vi "Drive Direction.vi"(6 "Wheel DevRef":T1={"DeviceStatus"={"status"=FALSE, "code"=0, "source"=""}, "Type"=enum."PWM", "PWM"={"PWM Channel"=enum."Invalid", "DeadBand"={"Name"="", "maxPositivePwm"=0, "minPositivePwm"=0, "centerPwm"=0, "maxNegativePwm"=0, "minNegativePwm"=0, "angularRange"=0}}, "CAN"={"Device Number"=0, "SetOutput VI Ref"=variant(refnum<vi> refnum), "GetOutput VI Ref"=variant(refnum<vi> refnum), "Enable VI Ref"=variant(refnum<vi> refnum), "Disable VI Ref"=variant(refnum<vi> refnum), "Data"=variant}, "Invert"=FALSE}, 7 "Swerve DevRef":T1={"DeviceStatus"={"status"=FALSE, "code"=0, "source"=""}, "Type"=enum."PWM", "PWM"={"PWM Channel"=enum."PWM 1", "DeadBand"={"Name"="", "maxPositivePwm"=0, "minPositivePwm"=0, "centerPwm"=0, "maxNegativePwm"=0, "minNegativePwm"=0, "angularRange"=0}}, "CAN"={"Device Number"=0, "SetOutput VI Ref"=variant(enum8{"Percent VBus", "Current", "Speed", "Position", "Voltage"} enum."Percent VBus"), "GetOutput VI Ref"=variant(refnum<k1> refnum), "Enable VI Ref"=variant(dbl 12.0), "Disable VI Ref"=variant(enum8{"Percent VBus", "Speed", "Position", "Slave", "Unchanged / Invalid", "Voltage Compensation", "Current", "Motion Profile"} enum."Percent VBus"), "Data"=variant}, "Invert"=FALSE}, 8 "error in":errorcluster, 9 "Wheel Power":dbl format="%#_13g", 10 "Desired direction (radians)":dbl=6.283185307179586 format="%#_13g") -> (0 "error out":errorcluster, 1 "Setpoint":dbl, 2 "Wheel Speed":dbl, 3 "Swerve Speed":dbl, 4 "Reverse?":bool)   [LabVIEW 2016]
uses:
  <vilib>/Rock Robotics/WPI/MotorControl/WPI_MotorControlDeviceRef.ctl
  <vilib>/Rock Robotics/WPI/MotorControl/WPI_MotorControlType.ctl
  <vilib>/Rock Robotics/SystemInterfaces/DIO/FPGA_DIOPWMChannel.ctl
  <vilib>/Rock Robotics/WPI/PWM/WPI_PWMDeadband.ctl
  Main/Robot Global Data.vi
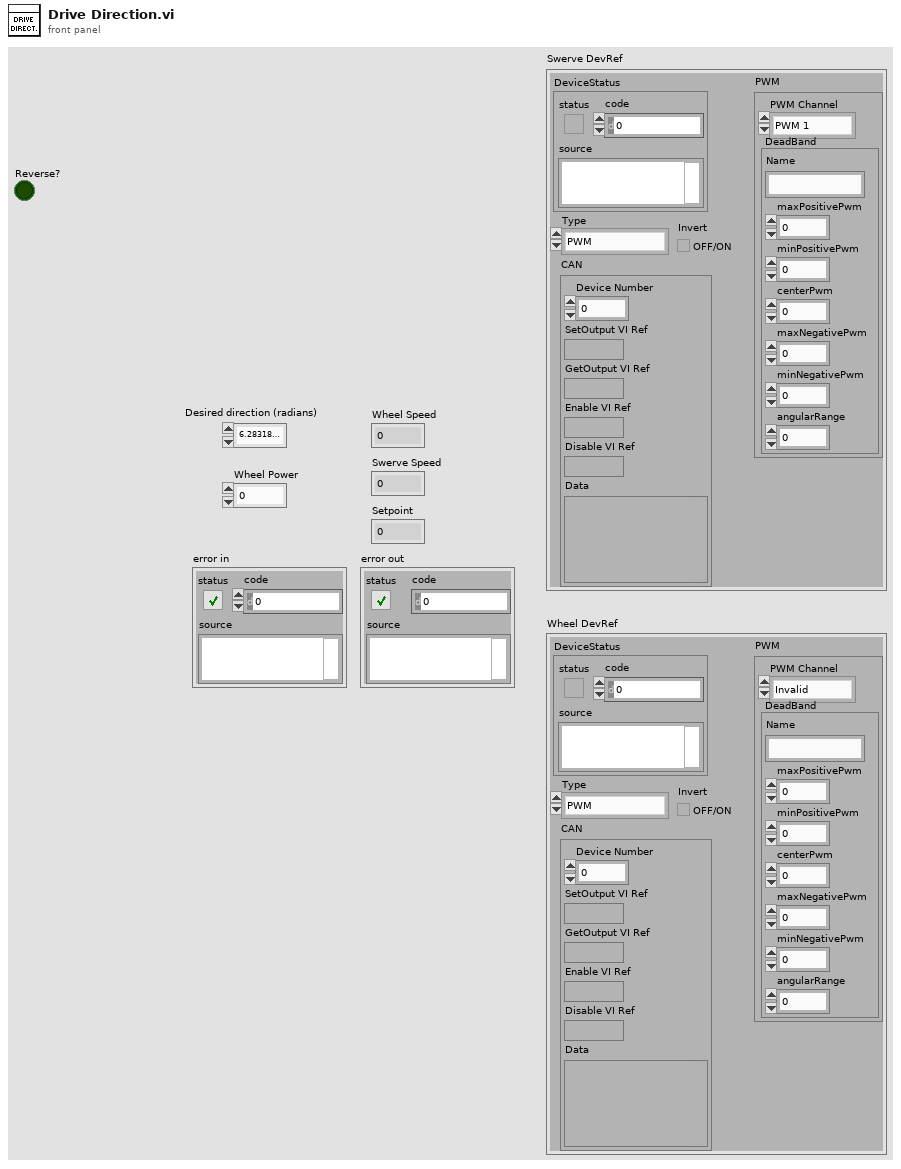
[diagram p1: front panel]
types:
  T1 = typedef "WPI_MotorControlDeviceRef.ctl" = cluster{"DeviceStatus":errorcluster, "Type":T2, "PWM":cluster{"PWM Channel":T3, "DeadBand":T4}, "CAN":cluster{"Device Number":u8, "SetOutput VI Ref":variant, "GetOutput VI Ref":variant, "Enable VI Ref":variant, "Disable VI Ref":variant, "Data":variant}, "Invert":bool}
  T2 = typedef "WPI_MotorControlType.ctl" = enum16{"PWM", "CAN"}
  T3 = typedef "FPGA_DIOPWMChannel.ctl" = enum8{"PWM 0", "PWM 1", "PWM 2", "PWM 3", "PWM 4", "PWM 5", "PWM 6", "PWM 7", "PWM 8", "PWM 9", "PWM MXP 0", "PWM MXP 1", "PWM MXP 2", "PWM MXP 3", "PWM MXP 4", "PWM MXP 5", "PWM MXP 6", "PWM MXP 7", "PWM MXP 8", "PWM MXP 9", "Invalid"}
  T4 = typedef "WPI_PWMDeadband.ctl" = cluster{"Name":string, "maxPositivePwm":i32, "minPositivePwm":i32, "centerPwm":i32, "maxNegativePwm":i32, "minNegativePwm":i32, "angularRange":u16}
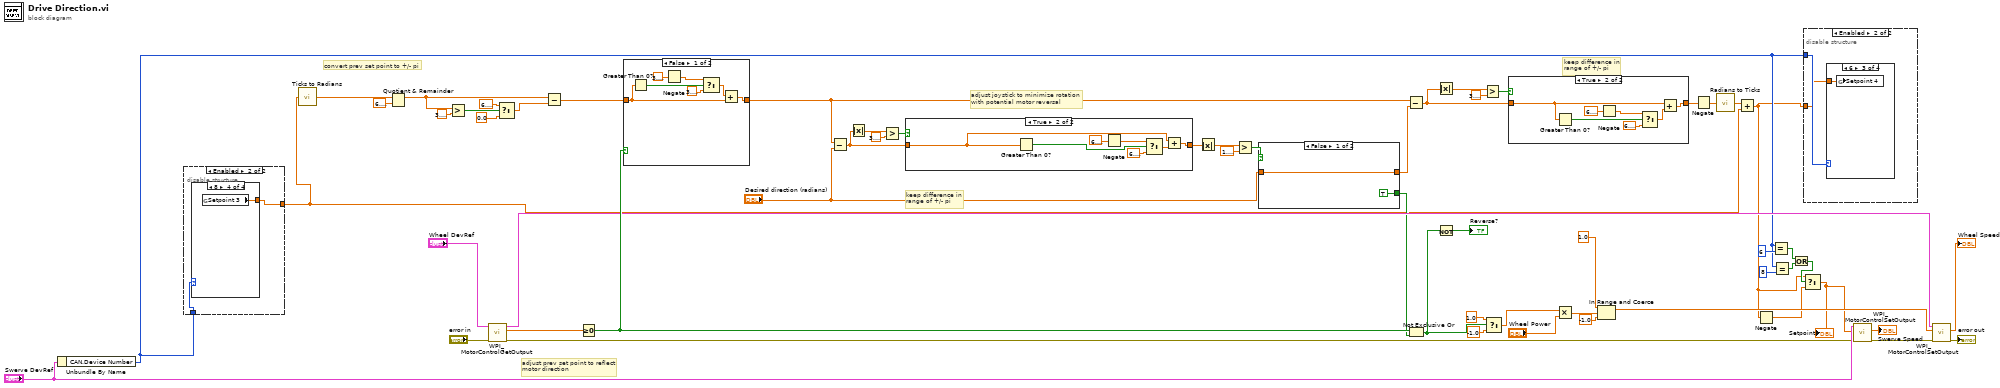
[diagram p0: block diagram]
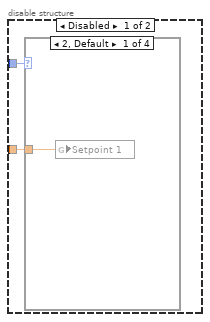
[diagram p2: hidden frame]
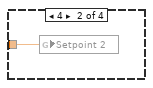
[diagram p3: hidden frame]
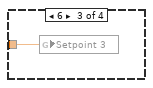
[diagram p4: hidden frame]
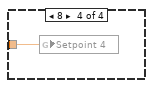
[diagram p5: hidden frame]
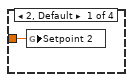
[diagram p6: hidden frame]
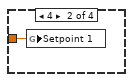
[diagram p7: hidden frame]
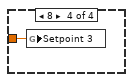
[diagram p8: hidden frame]
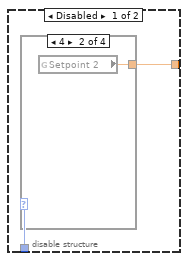
[diagram p9: hidden frame]
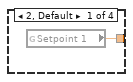
[diagram p10: hidden frame]
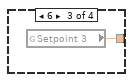
[diagram p11: hidden frame]
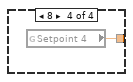
[diagram p12: hidden frame]
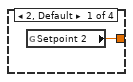
[diagram p13: hidden frame]
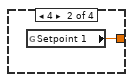
[diagram p14: hidden frame]
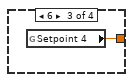
[diagram p15: hidden frame]
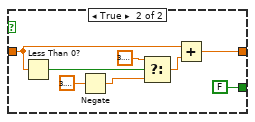
[diagram p17: hidden frame]
diagram:
  # "keep difference in\nrange of +/- pi"
  # "adjust joystick to minimize rotation\nwith potential motor reversal"
  # "keep difference in\nrange of +/- pi"
  # "adjust prev set point to reflect\nmotor direction"
  # "convert prev set point to +/- pi"
  n1 = Unbundle By Name("Swerve DevRef") -> ("CAN.Device Number"=w2:u8)
  n2 = disable-structure shown="Enabled" {
    disable-tunnel: w2 -> [w61 w67]
    disable-tunnel: [w60 w66] -> w22
    frame Disabled {
      n3 = case shown="4" w61 {
        tunnel: [w62 w63 w64 w65] -> w60
        frame 2, Default {
          n4 = global read "Robot Global Data.vi" "Setpoint 1"() -> (w62:dbl)
        }
        frame 4 {
          n5 = global read "Robot Global Data.vi" "Setpoint 2"() -> (w63:dbl)
        }
        frame 6 {
          n6 = global read "Robot Global Data.vi" "Setpoint 3"() -> (w64:dbl)
        }
        frame 8 {
          n7 = global read "Robot Global Data.vi" "Setpoint 4"() -> (w65:dbl)
        }
      }
    }
    frame Enabled {
      n8 = case shown="8" w67 {
        tunnel: [w68 w69 w70 w71] -> w66
        frame 2, Default {
          n9 = global read "Robot Global Data.vi" "Setpoint 2"() -> (w68:dbl)
        }
        frame 4 {
          n10 = global read "Robot Global Data.vi" "Setpoint 1"() -> (w69:dbl)
        }
        frame 6 {
          n11 = global read "Robot Global Data.vi" "Setpoint 4"() -> (w70:dbl)
        }
        frame 8 {
          n12 = global read "Robot Global Data.vi" "Setpoint 3"() -> (w71:dbl)
        }
      }
    }
  }
  n13 = call "Ticks to Radians.vi"("Ticks"=w22) -> ("Radians"=w47:dbl)
  n14 = Quotient & Remainder(x=w47, y=6.283185307179586) -> (x-y*floor(x/y)=w53:dbl)  [unwired: 1 out]
  n15 = Greater?(x=w53, y=3.141592653589793) -> (0:w57:bool)
  n16 = call <vilib>:"WPI_MotorControlGetOutput.vi"("error in"="error in", "MotorControlDevRef"="Wheel DevRef") -> ("error out"=w20:errorcluster, "Output"=w41:dbl, "MotorControlDevRef"=w40:T1)  [unwired: 7 in]
  n17 = Select(t=6.283185307179586, s=w57, f=0.0) -> (s? t:f=w54:dbl)
  n18 = Subtract(x=w53, y=w54) -> (x-y=w49:dbl)
  n19 = Greater Or Equal To 0?(x=w41) -> (x >= 0?=w48:bool)
  n20 = case shown="False" w48 {
    tunnel: w49 -> [w73 w79]
    tunnel: [w72 w79] -> w35
    frame False {
      n21 = Greater Than 0?(x=w73) -> (x > 0?=w78:bool)
      n22 = Negate(x=3.141592653589793) -> (-x=w77:dbl)
      n23 = Select(t=w77, s=w78, f=3.141592653589793) -> (s? t:f=w74:dbl)
      n24 = Add(x=w74, y=w73) -> (x+y=w72:dbl)
    }
    frame True {
    }
  }
  n25 = Subtract(x=w35, y="Desired direction (radians)") -> (x-y=w37:dbl)
  n26 = Absolute Value(x=w37) -> (abs(x)=w50:dbl)
  n27 = Greater?(x=w50, y=3.141592653589793) -> (0:w52:bool)
  n28 = case shown="True" w52 {
    tunnel: w37 -> [w80 w82]
    tunnel: [w80 w81] -> w36
    frame False {
    }
    frame True {
      n29 = Greater Than 0?(x=w82) -> (x > 0?=w87:bool)
      n30 = Negate(x=6.283185307179586) -> (-x=w84:dbl)
      n31 = Select(t=w84, s=w87, f=6.283185307179586) -> (s? t:f=w83:dbl)
      n32 = Add(x=w82, y=w83) -> (x+y=w81:dbl)
    }
  }
  n33 = Absolute Value(x=w36) -> (abs(x)=w17:dbl)
  n34 = Greater?(x=w17, y=1.5707963267948966) -> (0:w16:bool)
  n35 = case shown="False" w16 {
    tunnel: "Desired direction (radians)" -> [w89 w92]
    tunnel: [w89 w91] -> w34
    tunnel: [TRUE FALSE] -> w33
    frame False {
    }
    frame True {
      n36 = Less Than 0?(x=w92) -> (x < 0?=w97:bool)
      n37 = Negate(x=3.141592653589793) -> (-x=w94:dbl)
      n38 = Select(t=3.141592653589793, s=w97, f=w94) -> (s? t:f=w93:dbl)
      n39 = Add(x=w92, y=w93) -> (x+y=w91:dbl)
    }
  }
  n40 = Subtract(x=w35, y=w34) -> (x-y=w29:dbl)
  n41 = Not Exclusive Or(1:w33, 2:w48) -> (0:w46:bool)
  n42 = Absolute Value(x=w29) -> (abs(x)=w32:dbl)
  n43 = Not(x=w46) -> (.not. x?=→"Reverse?":bool)
  n44 = Greater?(x=w32, y=3.141592653589793) -> (0:w31:bool)
  n45 = Select(t=1.0, s=w46, f=-1.0 ("t")) -> (s? t:f=w43:dbl)
  n46 = case shown="True" w31 {
    tunnel: w29 -> [w98 w100]
    tunnel: [w98 w99] -> w28
    frame False {
    }
    frame True {
      n47 = Greater Than 0?(x=w100) -> (x > 0?=w105:bool)
      n48 = Negate(x=6.283185307179586) -> (-x=w103:dbl)
      n49 = Select(t=w103, s=w105, f=6.283185307179586) -> (s? t:f=w102:dbl)
      n50 = Add(x=w100, y=w102) -> (x+y=w99:dbl)
    }
  }
  n51 = Multiply(x=w43, y="Wheel Power") -> (x*y=w10:dbl)
  n52 = In Range and Coerce(upper limit=1.0, x=w10, lower limit=-1.0) -> (coerced(x)=w12:dbl)  [unwired: 1 out]
  n53 = Negate(x=w28) -> (-x=w23:dbl)
  n54 = call "Radians to Ticks.vi"("Radians"=w23) -> ("Ticks"=w27:dbl)
  n55 = Add(x=w27, y=w22) -> (x+y=w1:dbl)
  n56 = Negate(x=w1) -> (-x=w4:dbl)
  n57 = Equal?(x=w2, y=u8 6) -> (x = y?=w7:bool)
  n58 = Equal?(x=w2, y=u8 8) -> (x = y?=w6:bool)
  n59 = Or(x=w7, y=w6) -> (x .or. y?=w5:bool)
  n60 = disable-structure shown="Enabled" {
    disable-tunnel: w2 -> [w107 w113]
    disable-tunnel: w1 -> [w106 w112]
    frame Disabled {
      n61 = case shown="2, Default" w107 {
        tunnel: w106 -> [w108 w109 w110 w111]
        frame 2, Default {
          n62 = global write "Robot Global Data.vi" "Setpoint 1"(w108) -> ()
        }
        frame 4 {
          n63 = global write "Robot Global Data.vi" "Setpoint 2"(w109) -> ()
        }
        frame 6 {
          n64 = global write "Robot Global Data.vi" "Setpoint 3"(w110) -> ()
        }
        frame 8 {
          n65 = global write "Robot Global Data.vi" "Setpoint 4"(w111) -> ()
        }
      }
    }
    frame Enabled {
      n66 = case shown="6" w113 {
        tunnel: w112 -> [w114 w115 w116 w117]
        frame 2, Default {
          n67 = global write "Robot Global Data.vi" "Setpoint 2"(w114) -> ()
        }
        frame 4 {
          n68 = global write "Robot Global Data.vi" "Setpoint 1"(w115) -> ()
        }
        frame 6 {
          n69 = global write "Robot Global Data.vi" "Setpoint 4"(w116) -> ()
        }
        frame 8 {
          n70 = global write "Robot Global Data.vi" "Setpoint 3"(w117) -> ()
        }
      }
    }
  }
  n71 = Select(t=w1, s=w5, f=w4) -> (s? t:f=w3:dbl)
  "Setpoint" <- w3
  n72 = call <vilib>:"WPI_MotorControlSetOutput.vi"("error in (no error)"=w20, "Output"=w3, "MotorControlDevRef"="Swerve DevRef") -> ("error out"=w18:errorcluster, "Motor Output"=→"Swerve Speed":dbl)  [unwired: 6 in, 1 out]
  n73 = call <vilib>:"WPI_MotorControlSetOutput.vi"("error in (no error)"=w18, "Output"=w12, "MotorControlDevRef"=w40) -> ("error out"=→"error out":errorcluster, "Motor Output"=→"Wheel Speed":dbl)  [unwired: 6 in, 1 out]
